vi "Write_Flatten.vi"(8 "error in":errorcluster, 10 "ChillerProducerChannels":T1, 11 "ChillerNew.lvclass":refnum<class "ChillerNew.lvclass">) -> (0 "error out":errorcluster, 3 "output cluster":refnum<class "ChillerNew.lvclass">)   [LabVIEW 2023, in "ChillerNew.lvclass"]
uses:
  ChillerNew.lvclass
  ChillerNew.lvclass/ChillerNew.ctl
  0d9857a9-8196-4fa2-a65b-709d35856b1d.vi
  0d9857a9-8196-4fa2-a65b-709d35856b1d.vi/4bc1c15b-36ab-481f-b8dd-c64075ce723a.vi
  0d9857a9-8196-4fa2-a65b-709d35856b1d.vi/d83cb72b-7713-41fc-a3d1-682de79cf574.vi
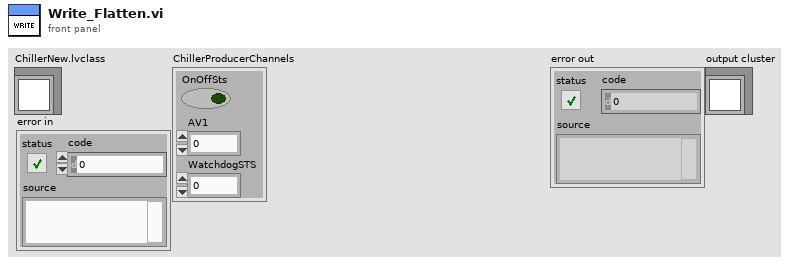
[diagram p1: front panel]
types:
  T1 = cluster{"OnOffSts":bool, "AV1":dbl, "WatchdogSTS":i32}
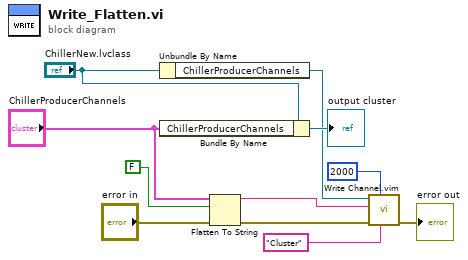
[diagram p0: block diagram]
diagram:
  n1 = Unbundle By Name("ChillerNew.lvclass") -> ("ChillerProducerChannels"=w8:refnum<k21>)
  n2 = Bundle By Name(cluster="ChillerNew.lvclass", "ChillerProducerChannels"="ChillerProducerChannels") -> (→"output cluster":refnum<class "ChillerNew.lvclass">)
  n3 = Flatten To String(anything="ChillerProducerChannels", prepend array or string size? (T)=FALSE, error in (no error)="error in") -> (data string=w3:string, error out=w1:errorcluster)  [unwired: 1 in, 1 out]
  n4 = call "Write Channel.vim"("Channel Type Description"="Cluster", "Timeout (ms)"=2000, "error in"=w1, "Data in"=w3, "ADAS HIL Channel in"=w8) -> ("error out"=→"error out":errorcluster)  [unwired: 4 in, 2 out]
